vi "REPORT.init test.vi"(10 "Test OUT 2":T1={"Config HW"={"VISA Rigol DP832"="USB0::0x1AB1::0x0E11::DP8C191500901::INSTR", "Config Rigol DP832"=[{"Channel"=0, "V Limit"=5.5, "I Limit"=0.5, "V Out"=5.0}, {"Channel"=1, "V Limit"=5.5, "I Limit"=0.8, "V Out"=5.0}, {"Channel"=2, "V Limit"=5.5, "I Limit"=0.2, "V Out"=0.0}], "CTA Test#"="CTA013 A", "FT_Handle"=432866568, "Espera acceso FT"=10, "VISA Tek MDO3104"="Rigol_DP832", "VISA Key 81160A"="Rigol_DP832"}, "Config Test"=[{"Vasic"=2.8, "Global Reset"=FALSE, "Test Register?"=FALSE, "Test ADC?"=FALSE, "Test ADC"={"Repeats ADC"=100, "Max Desviation"=0.1}, "Limits ADC"={"Low"=[1.9, 1.3, 0.65, 0.0, 1.6, 1.4, 1.4, 0.9, 2.1, 0.85, 1.9], "High"=[2.1, 1.5, 0.85, 0.1, 1.4, 1.2, 1.2, 0.7, 1.9, 0.65, 1.7]}, "Test Max PN Min NP?"=FALSE, "Limits Max PN Min NP"={"Max P Upper"=2.177000045776367, "Min P Upper"=1.474, "Max N Upper"=1.475, "Min N Upper"=0.818, "Max P Lower"=1.888, "Min P Lower "=1.321, "Max N Lower"=1.322, "Min N Lower"=0.73}, "Test Rate Scan?"=FALSE, "Vin Rate Scan"=[], "Limits Rate Scan"={"High"=[0.15, 0.242, 0.331, 0.425, 0.512, 0.6, 0.688, 0.774, 0.847, 0.91], "Low"=[0.021, 0.11, 0.189, 0.27, 0.347, 0.421, 0.487, 0.551, 0.601, 0.635]}, "Test Rate Scan Adders?"=FALSE, "Vin Rate Adders"=[], "Limits Rate Scan adders"={"High"=[], "Low"=[]}, "Test offset analog?"=FALSE, "Lim Offset Analog"={"Max Analog"=0.05, "Min Analog"=-0.05}, "Test offset digital?"=FALSE, "Lim offset Dig"={"Max Dig"=0.05}, "Vasic real f.a."=2.8, "IBIAS"=FALSE, "VALUE IBIAS"=63}, {"Vasic"=2.8, "Global Reset"=FALSE, "Test Register?"=FALSE, "Test ADC?"=FALSE, "Test ADC"={"Repeats ADC"=100, "Max Desviation"=0.1}, "Limits ADC"={"Low"=[1.9, 1.3, 0.65, 0.0, 1.6, 1.4, 1.4, 0.9, 2.1, 0.85, 1.9], "High"=[2.1, 1.5, 0.85, 0.1, 1.4, 1.2, 1.2, 0.7, 1.9, 0.65, 1.7]}, "Test Max PN Min NP?"=FALSE, "Limits Max PN Min NP"={"Max P Upper"=2.177000045776367, "Min P Upper"=1.474, "Max N Upper"=1.475, "Min N Upper"=0.818, "Max P Lower"=1.888, "Min P Lower "=1.321, "Max N Lower"=1.322, "Min N Lower"=0.73}, "Test Rate Scan?"=FALSE, "Vin Rate Scan"=[], "Limits Rate Scan"={"High"=[0.15, 0.242, 0.331, 0.425, 0.512, 0.6, 0.688, 0.774, 0.847, 0.91], "Low"=[0.021, 0.11, 0.189, 0.27, 0.347, 0.421, 0.487, 0.551, 0.601, 0.635]}, "Test Rate Scan Adders?"=FALSE, "Vin Rate Adders"=[], "Limits Rate Scan adders"={"High"=[], "Low"=[]}, "Test offset analog?"=FALSE, "Lim Offset Analog"={"Max Analog"=0.05, "Min Analog"=-0.05}, "Test offset digital?"=FALSE, "Lim offset Dig"={"Max Dig"=0.05}, "Vasic real f.a."=2.8, "IBIAS"=FALSE, "VALUE IBIAS"=63}, {"Vasic"=2.8, "Global Reset"=FALSE, "Test Register?"=FALSE, "Test ADC?"=FALSE, "Test ADC"={"Repeats ADC"=100, "Max Desviation"=0.1}, "Limits ADC"={"Low"=[1.9, 1.3, 0.65, 0.0, 1.6, 1.4, 1.4, 0.9, 2.1, 0.85, 1.9], "High"=[2.1, 1.5, 0.85, 0.1, 1.4, 1.2, 1.2, 0.7, 1.9, 0.65, 1.7]}, "Test Max PN Min NP?"=FALSE, "Limits Max PN Min NP"={"Max P Upper"=2.177000045776367, "Min P Upper"=1.474, "Max N Upper"=1.475, "Min N Upper"=0.818, "Max P Lower"=1.888, "Min P Lower "=1.321, "Max N Lower"=1.322, "Min N Lower"=0.73}, "Test Rate Scan?"=FALSE, "Vin Rate Scan"=[], "Limits Rate Scan"={"High"=[0.15, 0.242, 0.331, 0.425, 0.512, 0.6, 0.688, 0.774, 0.847, 0.91], "Low"=[0.021, 0.11, 0.189, 0.27, 0.347, 0.421, 0.487, 0.551, 0.601, 0.635]}, "Test Rate Scan Adders?"=FALSE, "Vin Rate Adders"=[], "Limits Rate Scan adders"={"High"=[], "Low"=[]}, "Test offset analog?"=FALSE, "Lim Offset Analog"={"Max Analog"=0.05, "Min Analog"=-0.05}, "Test offset digital?"=FALSE, "Lim offset Dig"={"Max Dig"=0.05}, "Vasic real f.a."=2.8, "IBIAS"=FALSE, "VALUE IBIAS"=63}, {"Vasic"=2.8, "Global Reset"=FALSE, "Test Register?"=FALSE, "Test ADC?"=FALSE, "Test ADC"={"Repeats ADC"=100, "Max Desviation"=0.1}, "Limits ADC"={"Low"=[1.9, 1.3, 0.65, 0.0, 1.6, 1.4, 1.4, 0.9, 2.1, 0.85, 1.9], "High"=[2.1, 1.5, 0.85, 0.1, 1.4, 1.2, 1.2, 0.7, 1.9, 0.65, 1.7]}, "Test Max PN Min NP?"=FALSE, "Limits Max PN Min NP"={"Max P Upper"=2.177000045776367, "Min P Upper"=1.474, "Max N Upper"=1.475, "Min N Upper"=0.818, "Max P Lower"=1.888, "Min P Lower "=1.321, "Max N Lower"=1.322, "Min N Lower"=0.73}, "Test Rate Scan?"=FALSE, "Vin Rate Scan"=[], "Limits Rate Scan"={"High"=[0.15, 0.242, 0.331, 0.425, 0.512, 0.6, 0.688, 0.774, 0.847, 0.91], "Low"=[0.021, 0.11, 0.189, 0.27, 0.347, 0.421, 0.487, 0.551, 0.601, 0.635]}, "Test Rate Scan Adders?"=FALSE, "Vin Rate Adders"=[], "Limits Rate Scan adders"={"High"=[], "Low"=[]}, "Test offset analog?"=FALSE, "Lim Offset Analog"={"Max Analog"=0.05, "Min Analog"=-0.05}, "Test offset digital?"=FALSE, "Lim offset Dig"={"Max Dig"=0.05}, "Vasic real f.a."=2.8, "IBIAS"=FALSE, "VALUE IBIAS"=63}], "Result"=[{"Vasic Volt"=0, "Test Registros"={"Default Register OK"=FALSE, "Pattern Default"=[], "Read Default"=[], "W/R Register OK"=FALSE, "Pattern W/R"=[], "Read W/R"=[]}, "Test Dacs"={"Desviacion OK"=FALSE, "Means"=[], "Deviations"=[], "Desviations OK"=[], "Means OK"=[], "Graph Histogram"=[]}, "Test Max-Min PN"={"Max P Mini N OK"=FALSE, "PTHT Max P Min N"=[], "PTHT Max P Min N OK"=[], "NTHT Max P Min N"=[], "NTHT Max P Min N OK"=[], "Min P Max N OK"=FALSE, "PTHT Max N Min P"=[], "PTHT Max N Min P OK"=[], "NTHT Max N Min P"=[], "NTHT Max N Min P OK"=[], "Ref"=[]}, "Test Rate Scan"={"Rate Scan OK"=FALSE, "DAC TH0,TH1,TH2"=[], "Volt HLTH"=[], "Rate HLTH OK"=[], "DAC TH3,TH4,TH5"=[], "Volt LLTH"=[], "Rate LLTH 2 OK"=[], "Scaler 0"=[], "Ref"=[], "OFFSET HLTH"=[], "OFFSET LLTH"=[], "Real Voltage"=[]}, "Test Rate Scan adders"={"Rate Scan Adders OK"=FALSE, "DAC TH0,TH1,TH2"=[], "Volt HLTH"=[], "Add HLTH OK"=[], "DAC TH3,TH4,TH5"=[], "Volt LLTH"=[], "Add LLTH 2 OK"=[], "Scaler 0"=[], "Ref"=[], "OFFSET HLTH"=[], "OFFSET LLTH"=[], "Real Voltage"=[]}, "Test Offset Analog"={"Offset Analog OK"=FALSE, "V ADDOUT"=[], "Offset OK"=[], "Ref"=[]}, "Test Offset Digital"={"Offset Digital OK"=FALSE, "SCALER 1 START"=[], "SCALER 1 STOP"=[], "THX START"=[], "THX STOP"=[], "VHLTH START"=[], "VHLTH STOP"=[], "Index 1 Start"=[], "index 1 Stop"=[], "SCALER 2 START"=[], "SCALER 2 STOP"=[], "THX+3 START"=[], "THX+3 STOP"=[], "VLLTH START"=[], "VLLTH STOP"=[], "Index 2 Start"=[], "index 2 Stop"=[], "Dig HLTH OK"=[], "Dig LLTH 2 OK"=[], "Ref"=[]}, "info hardware"={"Iout V1"=0.0, "Iout V2"=0.0, "Iout V3"=0.0, "Vout V1"=0.0, "Vout V2"=0.0, "Vout V3"=0.0, "Temp"=0.0}, "Test Offset Analog add"={"Offset Analog add OK"=FALSE, "V ADDOUT add"=[], "Offset add OK"=[], "Ref add"=[]}, "info temp"={"T Asic Registers"=0.0, "T Board Test. ADC"=0.0, "T Asic Max Min N P"=0.0, "T Adc count"=0.0, "T Asic Digital Offset"=0.0, "T Asic Analog Offset"=0.0, "T Asic Analog add"=0.0, "T Asic Rate Scan"=0.0, "T Asic Rate Scan Adders"=0.0, "T Final"=0.0}}, {"Vasic Volt"=0, "Test Registros"={"Default Register OK"=FALSE, "Pattern Default"=[], "Read Default"=[], "W/R Register OK"=FALSE, "Pattern W/R"=[], "Read W/R"=[]}, "Test Dacs"={"Desviacion OK"=FALSE, "Means"=[], "Deviations"=[], "Desviations OK"=[], "Means OK"=[], "Graph Histogram"=[]}, "Test Max-Min PN"={"Max P Mini N OK"=FALSE, "PTHT Max P Min N"=[], "PTHT Max P Min N OK"=[], "NTHT Max P Min N"=[], "NTHT Max P Min N OK"=[], "Min P Max N OK"=FALSE, "PTHT Max N Min P"=[], "PTHT Max N Min P OK"=[], "NTHT Max N Min P"=[], "NTHT Max N Min P OK"=[], "Ref"=[]}, "Test Rate Scan"={"Rate Scan OK"=FALSE, "DAC TH0,TH1,TH2"=[], "Volt HLTH"=[], "Rate HLTH OK"=[], "DAC TH3,TH4,TH5"=[], "Volt LLTH"=[], "Rate LLTH 2 OK"=[], "Scaler 0"=[], "Ref"=[], "OFFSET HLTH"=[], "OFFSET LLTH"=[], "Real Voltage"=[]}, "Test Rate Scan adders"={"Rate Scan Adders OK"=FALSE, "DAC TH0,TH1,TH2"=[], "Volt HLTH"=[], "Add HLTH OK"=[], "DAC TH3,TH4,TH5"=[], "Volt LLTH"=[], "Add LLTH 2 OK"=[], "Scaler 0"=[], "Ref"=[], "OFFSET HLTH"=[], "OFFSET LLTH"=[], "Real Voltage"=[]}, "Test Offset Analog"={"Offset Analog OK"=FALSE, "V ADDOUT"=[], "Offset OK"=[], "Ref"=[]}, "Test Offset Digital"={"Offset Digital OK"=FALSE, "SCALER 1 START"=[], "SCALER 1 STOP"=[], "THX START"=[], "THX STOP"=[], "VHLTH START"=[], "VHLTH STOP"=[], "Index 1 Start"=[], "index 1 Stop"=[], "SCALER 2 START"=[], "SCALER 2 STOP"=[], "THX+3 START"=[], "THX+3 STOP"=[], "VLLTH START"=[], "VLLTH STOP"=[], "Index 2 Start"=[], "index 2 Stop"=[], "Dig HLTH OK"=[], "Dig LLTH 2 OK"=[], "Ref"=[]}, "info hardware"={"Iout V1"=0.0, "Iout V2"=0.0, "Iout V3"=0.0, "Vout V1"=0.0, "Vout V2"=0.0, "Vout V3"=0.0, "Temp"=0.0}, "Test Offset Analog add"={"Offset Analog add OK"=FALSE, "V ADDOUT add"=[], "Offset add OK"=[], "Ref add"=[]}, "info temp"={"T Asic Registers"=0.0, "T Board Test. ADC"=0.0, "T Asic Max Min N P"=0.0, "T Adc count"=0.0, "T Asic Digital Offset"=0.0, "T Asic Analog Offset"=0.0, "T Asic Analog add"=0.0, "T Asic Rate Scan"=0.0, "T Asic Rate Scan Adders"=0.0, "T Final"=0.0}}, {"Vasic Volt"=0, "Test Registros"={"Default Register OK"=FALSE, "Pattern Default"=[], "Read Default"=[], "W/R Register OK"=FALSE, "Pattern W/R"=[], "Read W/R"=[]}, "Test Dacs"={"Desviacion OK"=FALSE, "Means"=[], "Deviations"=[], "Desviations OK"=[], "Means OK"=[], "Graph Histogram"=[]}, "Test Max-Min PN"={"Max P Mini N OK"=FALSE, "PTHT Max P Min N"=[], "PTHT Max P Min N OK"=[], "NTHT Max P Min N"=[], "NTHT Max P Min N OK"=[], "Min P Max N OK"=FALSE, "PTHT Max N Min P"=[], "PTHT Max N Min P OK"=[], "NTHT Max N Min P"=[], "NTHT Max N Min P OK"=[], "Ref"=[]}, "Test Rate Scan"={"Rate Scan OK"=FALSE, "DAC TH0,TH1,TH2"=[], "Volt HLTH"=[], "Rate HLTH OK"=[], "DAC TH3,TH4,TH5"=[], "Volt LLTH"=[], "Rate LLTH 2 OK"=[], "Scaler 0"=[], "Ref"=[], "OFFSET HLTH"=[], "OFFSET LLTH"=[], "Real Voltage"=[]}, "Test Rate Scan adders"={"Rate Scan Adders OK"=FALSE, "DAC TH0,TH1,TH2"=[], "Volt HLTH"=[], "Add HLTH OK"=[], "DAC TH3,TH4,TH5"=[], "Volt LLTH"=[], "Add LLTH 2 OK"=[], "Scaler 0"=[], "Ref"=[], "OFFSET HLTH"=[], "OFFSET LLTH"=[], "Real Voltage"=[]}, "Test Offset Analog"={"Offset Analog OK"=FALSE, "V ADDOUT"=[], "Offset OK"=[], "Ref"=[]}, "Test Offset Digital"={"Offset Digital OK"=FALSE, "SCALER 1 START"=[], "SCALER 1 STOP"=[], "THX START"=[], "THX STOP"=[], "VHLTH START"=[], "VHLTH STOP"=[], "Index 1 Start"=[], "index 1 Stop"=[], "SCALER 2 START"=[], "SCALER 2 STOP"=[], "THX+3 START"=[], "THX+3 STOP"=[], "VLLTH START"=[], "VLLTH STOP"=[], "Index 2 Start"=[], "index 2 Stop"=[], "Dig HLTH OK"=[], "Dig LLTH 2 OK"=[], "Ref"=[]}, "info hardware"={"Iout V1"=0.0, "Iout V2"=0.0, "Iout V3"=0.0, "Vout V1"=0.0, "Vout V2"=0.0, "Vout V3"=0.0, "Temp"=0.0}, "Test Offset Analog add"={"Offset Analog add OK"=FALSE, "V ADDOUT add"=[], "Offset add OK"=[], "Ref add"=[]}, "info temp"={"T Asic Registers"=0.0, "T Board Test. ADC"=0.0, "T Asic Max Min N P"=0.0, "T Adc count"=0.0, "T Asic Digital Offset"=0.0, "T Asic Analog Offset"=0.0, "T Asic Analog add"=0.0, "T Asic Rate Scan"=0.0, "T Asic Rate Scan Adders"=0.0, "T Final"=0.0}}, {"Vasic Volt"=0, "Test Registros"={"Default Register OK"=FALSE, "Pattern Default"=[], "Read Default"=[], "W/R Register OK"=FALSE, "Pattern W/R"=[], "Read W/R"=[]}, "Test Dacs"={"Desviacion OK"=FALSE, "Means"=[], "Deviations"=[], "Desviations OK"=[], "Means OK"=[], "Graph Histogram"=[]}, "Test Max-Min PN"={"Max P Mini N OK"=FALSE, "PTHT Max P Min N"=[], "PTHT Max P Min N OK"=[], "NTHT Max P Min N"=[], "NTHT Max P Min N OK"=[], "Min P Max N OK"=FALSE, "PTHT Max N Min P"=[], "PTHT Max N Min P OK"=[], "NTHT Max N Min P"=[], "NTHT Max N Min P OK"=[], "Ref"=[]}, "Test Rate Scan"={"Rate Scan OK"=FALSE, "DAC TH0,TH1,TH2"=[], "Volt HLTH"=[], "Rate HLTH OK"=[], "DAC TH3,TH4,TH5"=[], "Volt LLTH"=[], "Rate LLTH 2 OK"=[], "Scaler 0"=[], "Ref"=[], "OFFSET HLTH"=[], "OFFSET LLTH"=[], "Real Voltage"=[]}, "Test Rate Scan adders"={"Rate Scan Adders OK"=FALSE, "DAC TH0,TH1,TH2"=[], "Volt HLTH"=[], "Add HLTH OK"=[], "DAC TH3,TH4,TH5"=[], "Volt LLTH"=[], "Add LLTH 2 OK"=[], "Scaler 0"=[], "Ref"=[], "OFFSET HLTH"=[], "OFFSET LLTH"=[], "Real Voltage"=[]}, "Test Offset Analog"={"Offset Analog OK"=FALSE, "V ADDOUT"=[], "Offset OK"=[], "Ref"=[]}, "Test Offset Digital"={"Offset Digital OK"=FALSE, "SCALER 1 START"=[], "SCALER 1 STOP"=[], "THX START"=[], "THX STOP"=[], "VHLTH START"=[], "VHLTH STOP"=[], "Index 1 Start"=[], "index 1 Stop"=[], "SCALER 2 START"=[], "SCALER 2 STOP"=[], "THX+3 START"=[], "THX+3 STOP"=[], "VLLTH START"=[], "VLLTH STOP"=[], "Index 2 Start"=[], "index 2 Stop"=[], "Dig HLTH OK"=[], "Dig LLTH 2 OK"=[], "Ref"=[]}, "info hardware"={"Iout V1"=0.0, "Iout V2"=0.0, "Iout V3"=0.0, "Vout V1"=0.0, "Vout V2"=0.0, "Vout V3"=0.0, "Temp"=0.0}, "Test Offset Analog add"={"Offset Analog add OK"=FALSE, "V ADDOUT add"=[], "Offset add OK"=[], "Ref add"=[]}, "info temp"={"T Asic Registers"=0.0, "T Board Test. ADC"=0.0, "T Asic Max Min N P"=0.0, "T Adc count"=0.0, "T Asic Digital Offset"=0.0, "T Asic Analog Offset"=0.0, "T Asic Analog add"=0.0, "T Asic Rate Scan"=0.0, "T Asic Rate Scan Adders"=0.0, "T Final"=0.0}}], "Execucion Test"={"Vasic Actual"=0}, "Config VGA"={"Theoretical Voltage"=[0.1, 0.2, 0.3, 0.4, 0.5, 0.6, 0.7, 0.8, 0.9, 1.0], "Real Voltage"=[0.10285, 0.20714, 0.29957, 0.40485, 0.49571, 0.60685, 0.69771, 0.80114, 0.89714, 0.99885], "Pulse Width"=57344, "Frecuency Pulse"=1000000.0, "VGA Gain"=[9, 16, 24, 34, 43, 52, 61, 72, 81, 93]}, "Test Info"={"Asic"="", "Operator"="", "Place"="", "Time start"=timestamp(0 s since 1904-01-01), "Time stop"=timestamp(0 s since 1904-01-01)}, "Info machine"={"SO"="", "SO Name"="", "SO Ver"="", "SO Build"="", "CPU"="", "APP"="", "APP YEAR"="", "APP ver"="", "APP User"="", "APP Serail"="", "MAC"=[], "PC NAME"=[], "PC IP"=[], "BIOS MANU"="", "BIOS NAME"="", "BIOS SERIAL"="", "BOARD MANU"="", "BOARD NAME"="", "BOARD SERIAL"="", "Driver Version"="", "Library Version"="", "FPGA Ver"=0, "ID CTA board"=0, "LAST BOOT"="", "LABVIEW Ver"=0}, "Partial Report"="", "CONFIG GEN"=[]} {"CONFIG GEN"."Vasic Theorical" min=1.0 max=1000000.0 step=1.0 format="%#_6pV"; "CONFIG GEN"."Frequency" min=0.001 max=333000000.0 step=1000.0 format="%#_6pHz"; "CONFIG GEN"."Leading Edge Time" min=1e-09 max=1.0 step=1e-10 format="%#_6ps"; "CONFIG GEN"."Trailing Edge Time" min=1e-09 max=1.0 step=1e-10 format="%#_6ps"; "CONFIG GEN"."Delay" min=0.0 max=1.0 step=1e-12 format="%#_6ps"; "CONFIG GEN"."Trigger Level Sync" items=["ECL", "TTL"]; "CONFIG GEN"."Trigger Sync Out" items=["AB"=3, "B"=2, "A"=1, "None"=0]; "CONFIG GEN"."Load" min=1.0 max=1000000.0 step=1.0 format="%#_6p"; "CONFIG GEN"."DC Offset" min=-10.0 max=10.0 step=0.1 format="%#_6pV"; "CONFIG GEN"."Amplitude" min=0.05 max=5.0 step=0.001 format="%#_6pV"; "CONFIG GEN"."Width Time" min=1.5e-09 max=1.0 step=1e-10 format="%#_6ps"; "CONFIG GEN"."Channel" items=["Channel1"=1, "Channel2"=2]; "Config VGA"."Theoretical Voltage" format="%1.4f"; "Config VGA"."VGA Gain" format="%02x"; "Config VGA"."Frecuency Pulse" format="%0_2p"; "Config VGA"."Pulse Width" format="%04x"; "Config VGA"."Real Voltage" format="%1.5f"; "Config Test"."VALUE IBIAS" max=63 step=1; "Config Test"."Vasic real f.a." min=2.8 max=3.8 step=0.01 format="%.2g"; "Config Test"."Limits Rate Scan adders"."Low" format="%1.3f"; "Config Test"."Limits Rate Scan adders"."High" format="%1.3f"; "Config Test"."Limits ADC"."High" format="%1.4f"; "Config Test"."Limits ADC"."Low" format="%1.3f"; "Config Test"."Lim offset Dig"."Max Dig" format="%.3g"; "Config Test"."Lim Offset Analog"."Min Analog" format="%.3g"; "Config Test"."Lim Offset Analog"."Max Analog" format="%.3g"; "Config Test"."Limits Rate Scan"."Low" format="%1.4f"; "Config Test"."Limits Rate Scan"."High" format="%1.3f"; "Config Test"."Limits Max PN Min NP"."Min P Upper" format="%.3g"; "Config Test"."Limits Max PN Min NP"."Min P Lower" format="%.3g"; "Config Test"."Limits Max PN Min NP"."Max N Lower" format="%.3g"; "Config Test"."Limits Max PN Min NP"."Max N Upper" format="%.3g"; "Config Test"."Limits Max PN Min NP"."Min N Lower" format="%.3g"; "Config Test"."Limits Max PN Min NP"."Min N Upper" format="%.3g"; "Config Test"."Limits Max PN Min NP"."Max P Upper" format="%.3g"; "Config Test"."Limits Max PN Min NP"."Max P Lower" format="%.3g"; "Config Test"."Vasic" min=2.8 max=3.8 step=0.01 format="%.2g"; "Config HW"."Config Rigol DP832"."Channel" items=["+30V Channel 1", "+30V Channel 2", "+5V Channel 3"]; "Config HW"."Config Rigol DP832"."V Limit" format="%.1g"; "Config HW"."Config Rigol DP832"."I Limit" format="%.1g"; "Config HW"."Config Rigol DP832"."V Out" format="%.1g"; "Result"."Test Registros"."Read W/R" format="%04x"; "Result"."Test Registros"."Pattern W/R" format="%04x"; "Result"."Test Registros"."Read Default" format="%04x"; "Result"."Test Registros"."Pattern Default" format="%04x"}, 11 "Text In":string) -> (1 "OK, Fault":string, 2 "OK, Fault 2":bool, 3 "Text Out":string)   [LabVIEW 2019]
uses:
  Test.ctl
  TEST.TEST CONFIG HW.ctl
  Rigol DP832/DP832_Control Channels.ctl
  TEST.TEST CONFIG TEST MATRIZ.ctl
  TEST.TEST CONFIG TEST.ctl
  TEST.TEST RESULT.ctl
  test_result fvasic.ctl
  TEST.TEST EXECUTION TEST.ctl
  TEST.TEST CONFIG VGA.ctl
  TEST.TEST TEST INFO.ctl
  TEST.TEST INFO PC.ctl
  GenPulse_configurar.ctl
panel:
  # "Modo 2\nModo 3\nModo 4\nModo 2\nModo 3\nModo 4"
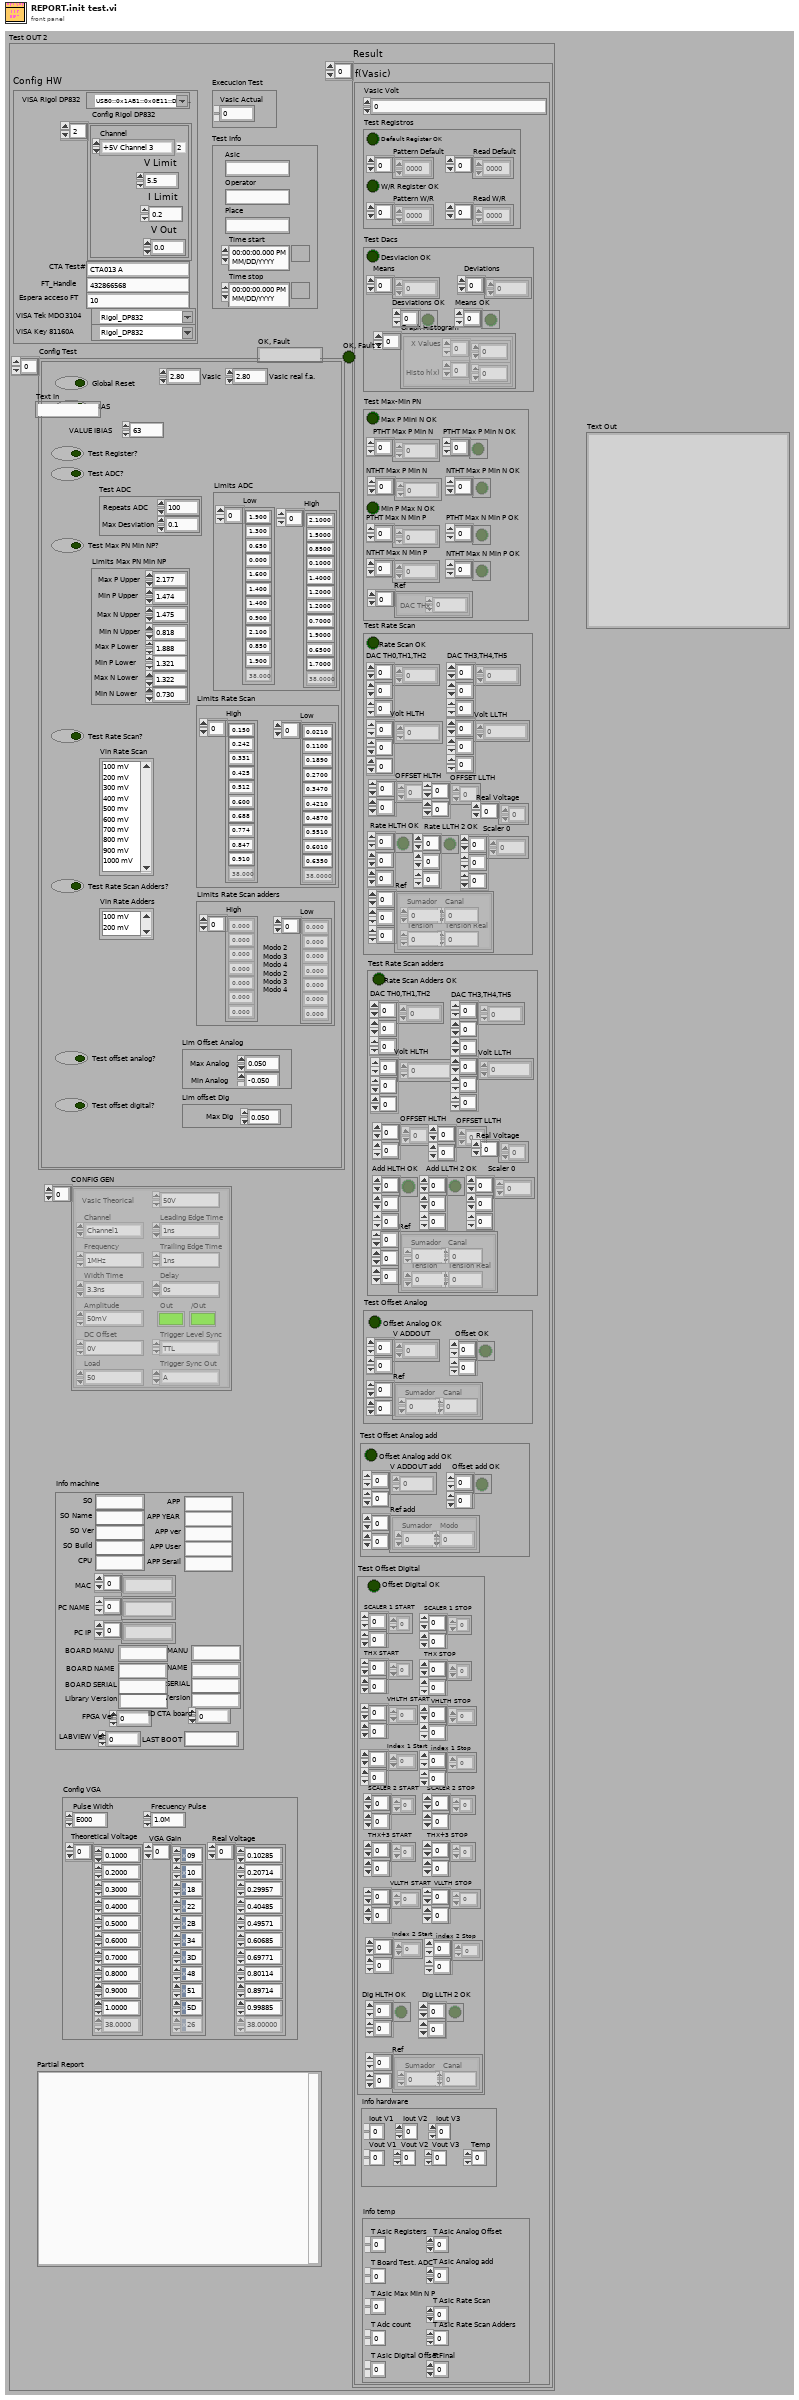
[diagram p1: front panel]
types:
  T1 = typedef "Test.ctl" = cluster{"Config HW":T2, "Config Test":T4, "Result":T6, "Execucion Test":T8, "Config VGA":T9, "Test Info":T10, "Info machine":T11, "Partial Report":string, "CONFIG GEN":T12[]}
  T2 = typedef "TEST.TEST CONFIG HW.ctl" = cluster{"VISA Rigol DP832":refnum<visa-resource-name>, "Config Rigol DP832":cluster{"Channel":T3, "V Limit":dbl, "I Limit":dbl, "V Out":dbl}[], "CTA Test#":string, "FT_Handle":u32, "Espera acceso FT":u32, "VISA Tek MDO3104":refnum<visa-resource-name>, "VISA Key 81160A":refnum<visa-resource-name>}
  T3 = typedef "DP832_Control Channels.ctl" = i32
  T4 = typedef "TEST.TEST CONFIG TEST MATRIZ.ctl" = T5[]
  T5 = typedef "TEST.TEST CONFIG TEST.ctl" = cluster{"Vasic":dbl, "Global Reset":bool, "Test Register?":bool, "Test ADC?":bool, "Test ADC":cluster{"Repeats ADC":i32, "Max Desviation":dbl}, "Limits ADC":cluster{"Low":dbl[], "High":dbl[]}, "Test Max PN Min NP?":bool, "Limits Max PN Min NP":cluster{"Max P Upper":dbl, "Min P Upper":dbl, "Max N Upper":dbl, "Min N Upper":dbl, "Max P Lower":dbl, "Min P Lower ":dbl, "Max N Lower":dbl, "Min N Lower":dbl}, "Test Rate Scan?":bool, "Vin Rate Scan":i32[], "Limits Rate Scan":cluster{"High":dbl[], "Low":dbl[]}, "Test Rate Scan Adders?":bool, "Vin Rate Adders":i32[], "Limits Rate Scan adders":cluster{"High":dbl[], "Low":dbl[]}, "Test offset analog?":bool, "Lim Offset Analog":cluster{"Max Analog":dbl, "Min Analog":dbl}, "Test offset digital?":bool, "Lim offset Dig":cluster{"Max Dig":dbl}, "Vasic real f.a.":dbl, "IBIAS":bool, "VALUE IBIAS":u8}
  T6 = typedef "TEST.TEST RESULT.ctl" = T7[]
  T7 = typedef "test_result fvasic.ctl" = cluster{"Vasic Volt":i32, "Test Registros":cluster{"Default Register OK":bool, "Pattern Default":u16[], "Read Default":u16[], "W/R Register OK":bool, "Pattern W/R":u16[], "Read W/R":u16[]}, "Test Dacs":cluster{"Desviacion OK":bool, "Means":dbl[], "Deviations":dbl[], "Desviations OK":bool[], "Means OK":bool[], "Graph Histogram":cluster{"X Values":dbl[], "Histo h(x)":i32[]}[]}, "Test Max-Min PN":cluster{"Max P Mini N OK":bool, "PTHT Max P Min N":dbl[], "PTHT Max P Min N OK":bool[], "NTHT Max P Min N":dbl[], "NTHT Max P Min N OK":bool[], "Min P Max N OK":bool, "PTHT Max N Min P":dbl[], "PTHT Max N Min P OK":bool[], "NTHT Max N Min P":dbl[], "NTHT Max N Min P OK":bool[], "Ref":cluster{"DAC THx":u8}[]}, "Test Rate Scan":cluster{"Rate Scan OK":bool, "DAC TH0,TH1,TH2":u16[][][], "Volt HLTH":dbl[][][], "Rate HLTH OK":bool[][][], "DAC TH3,TH4,TH5":u16[][][], "Volt LLTH":dbl[][][], "Rate LLTH 2 OK":bool[][][], "Scaler 0":u16[][][], "Ref":cluster{"Sumador":u8, "Canal":u8, "Tension":u8, "Tension Real":dbl}[][][], "OFFSET HLTH":dbl[][], "OFFSET LLTH":dbl[][], "Real Voltage":dbl[]}, "Test Rate Scan adders":cluster{"Rate Scan Adders OK":bool, "DAC TH0,TH1,TH2":u16[][][], "Volt HLTH":dbl[][][], "Add HLTH OK":bool[][][], "DAC TH3,TH4,TH5":u16[][][], "Volt LLTH":dbl[][][], "Add LLTH 2 OK":bool[][][], "Scaler 0":u16[][][], "Ref":cluster{"Sumador":u8, "Canal":u8, "Tension":u8, "Tension Real":dbl}[][][], "OFFSET HLTH":dbl[][], "OFFSET LLTH":dbl[][], "Real Voltage":dbl[]}, "Test Offset Analog":cluster{"Offset Analog OK":bool, "V ADDOUT":dbl[][], "Offset OK":bool[][], "Ref":cluster{"Sumador":u8, "Canal":u8}[][]}, "Test Offset Digital":cluster{"Offset Digital OK":bool, "SCALER 1 START":u16[][], "SCALER 1 STOP":u16[][], "THX START":u16[][], "THX STOP":u16[][], "VHLTH START":dbl[][], "VHLTH STOP":dbl[][], "Index 1 Start":i32[][], "index 1 Stop":i32[][], "SCALER 2 START":u16[][], "SCALER 2 STOP":u16[][], "THX+3 START":u16[][], "THX+3 STOP":u16[][], "VLLTH START":dbl[][], "VLLTH STOP":dbl[][], "Index 2 Start":i32[][], "index 2 Stop":i32[][], "Dig HLTH OK":bool[][], "Dig LLTH 2 OK":bool[][], "Ref":cluster{"Sumador":u8, "Canal":u8}[][]}, "info hardware":cluster{"Iout V1":dbl, "Iout V2":dbl, "Iout V3":dbl, "Vout V1":dbl, "Vout V2":dbl, "Vout V3":dbl, "Temp":dbl}, "Test Offset Analog add":cluster{"Offset Analog add OK":bool, "V ADDOUT add":dbl[][], "Offset add OK":bool[][], "Ref add":cluster{"Sumador":u8, "Modo":u8}[][]}, "info temp":cluster{"T Asic Registers":dbl, "T Board Test. ADC":dbl, "T Asic Max Min N P":dbl, "T Adc count":dbl, "T Asic Digital Offset":dbl, "T Asic Analog Offset":dbl, "T Asic Analog add":dbl, "T Asic Rate Scan":dbl, "T Asic Rate Scan Adders":dbl, "T Final":dbl}}
  T8 = typedef "TEST.TEST EXECUTION TEST.ctl" = cluster{"Vasic Actual":i32}
  T9 = typedef "TEST.TEST CONFIG VGA.ctl" = cluster{"Theoretical Voltage":dbl[], "Real Voltage":dbl[], "Pulse Width":u16, "Frecuency Pulse":dbl, "VGA Gain":u8[]}
  T10 = typedef "TEST.TEST TEST INFO.ctl" = cluster{"Asic":string, "Operator":string, "Place":string, "Time start":timestamp, "Time stop":timestamp}
  T11 = typedef "TEST.TEST INFO PC.ctl" = cluster{"SO":string, "SO Name":string, "SO Ver":string, "SO Build":string, "CPU":string, "APP":string, "APP YEAR":string, "APP ver":string, "APP User":string, "APP Serail":string, "MAC":string[], "PC NAME":string[], "PC IP":string[], "BIOS MANU":string, "BIOS NAME":string, "BIOS SERIAL":string, "BOARD MANU":string, "BOARD NAME":string, "BOARD SERIAL":string, "Driver Version":string, "Library Version":string, "FPGA Ver":u8, "ID CTA board":u64, "LAST BOOT":string, "LABVIEW Ver":u32}
  T12 = typedef "GenPulse_configurar.ctl" = cluster{"Channel":u16, "Frequency":dbl, "Width Time":dbl, "Amplitude":dbl, "DC Offset":dbl, "Load":dbl, "Leading Edge Time":dbl, "Trailing Edge Time":dbl, "Delay":dbl, "Out":bool, "/Out":bool, "Trigger Level Sync":u16, "Trigger Sync Out":u16, "Vasic Theorical":dbl}
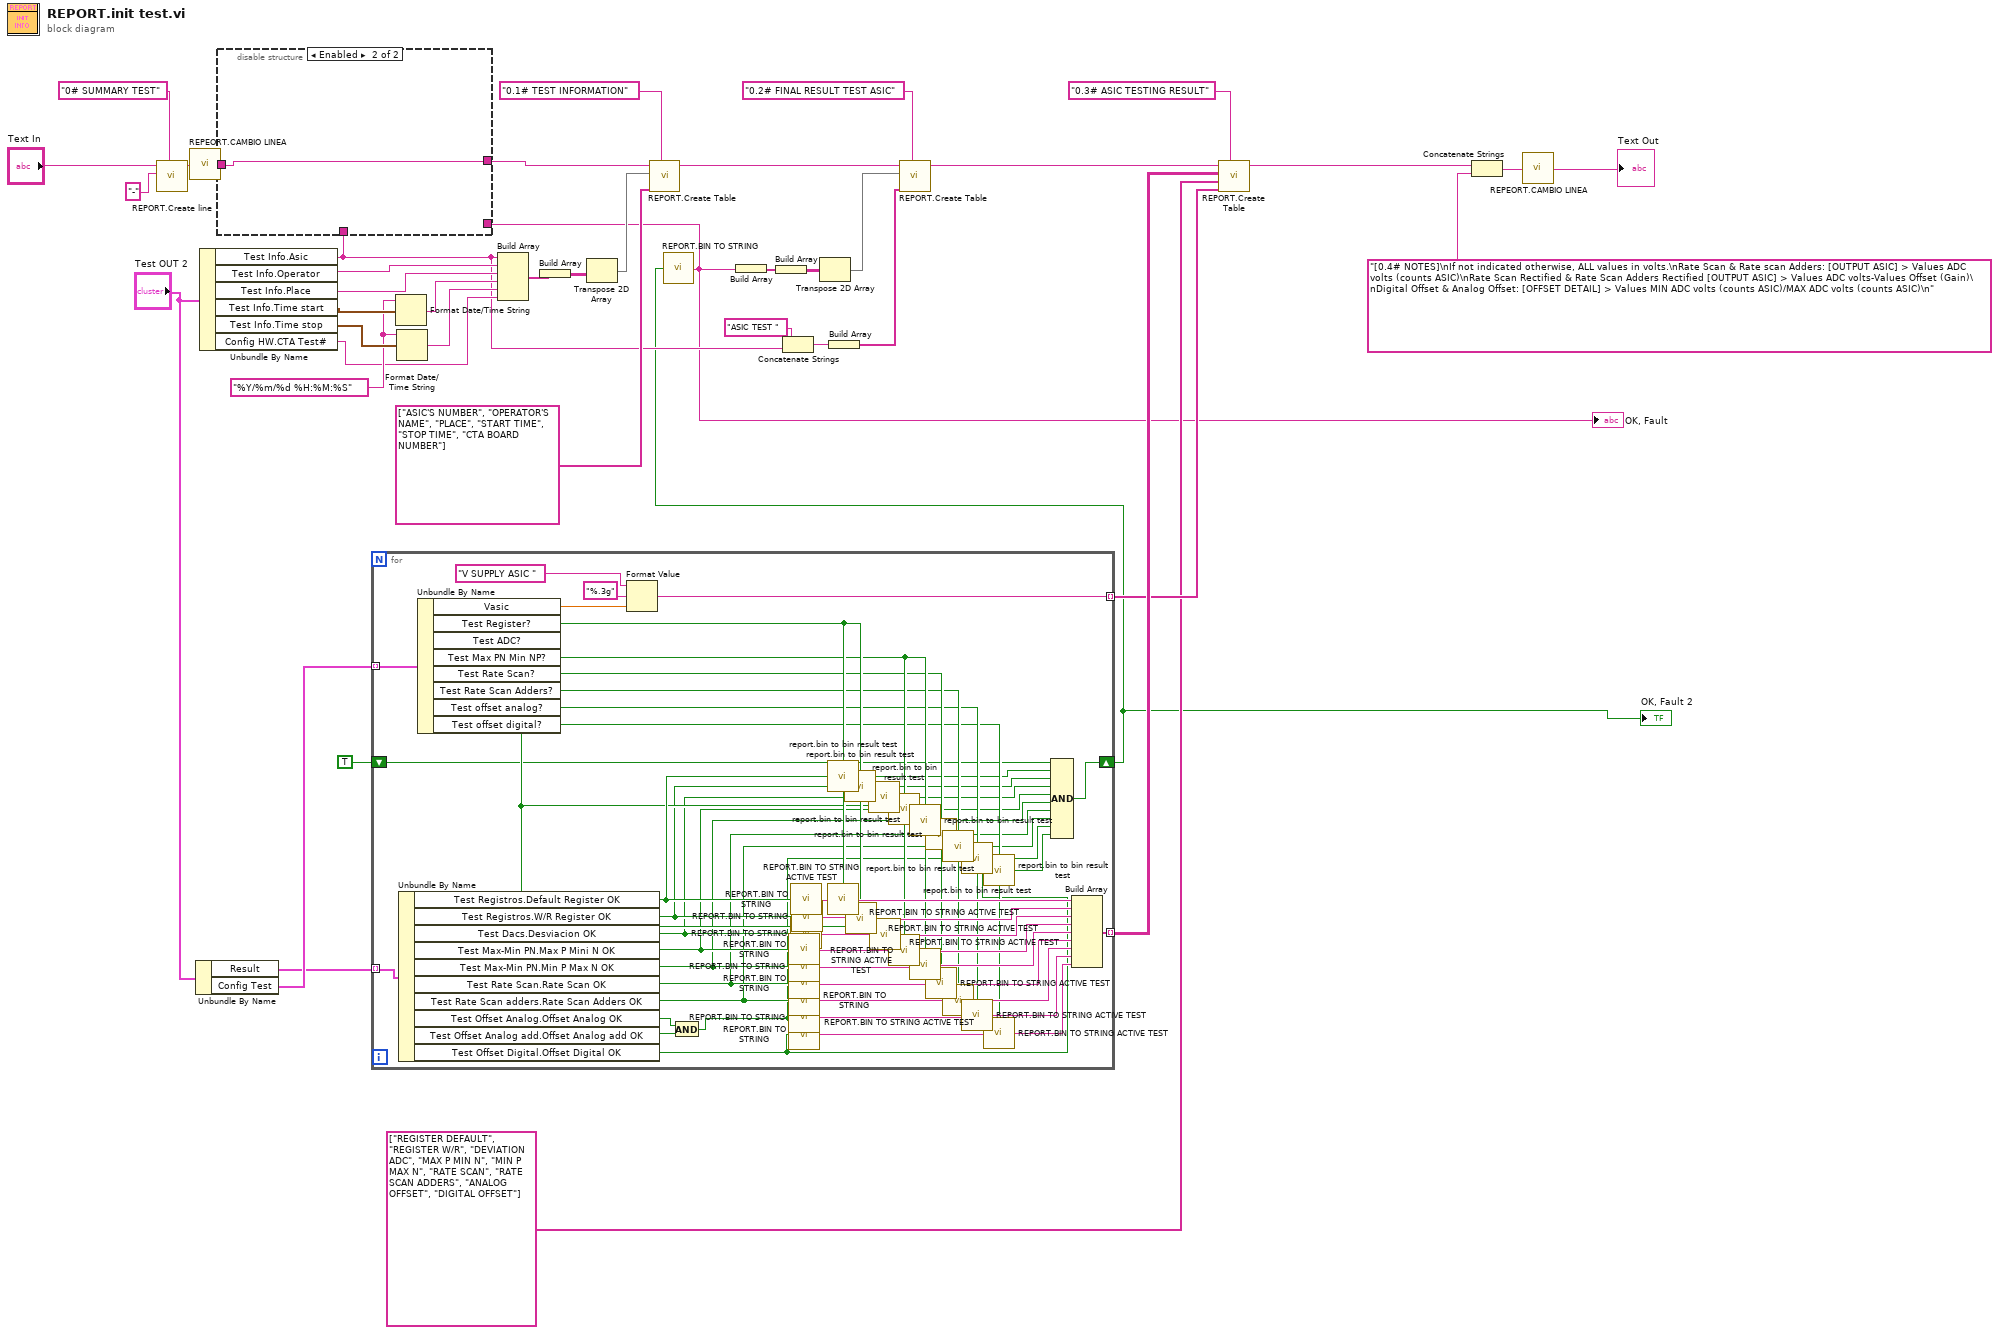
[diagram p0: block diagram]
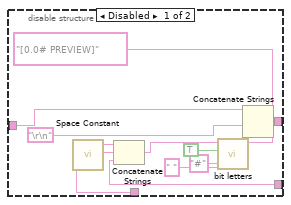
[diagram p2: hidden frame]
diagram:
  w38 = "%Y/%m/%d %H:%M:%S" ("time format string (%c)")
  n1 = call "REPORT.Create line.vi"("Secction"="0# SUMMARY TEST", "Char"="-", "Text In"="Text In") -> ("Text Out"=w28:string)  [unwired: 8 in]
  n2 = call "REPEORT.CAMBIO LINEA.vi"("Text Out"=w28) -> ("String"=w3:string)  [unwired: 8 in]
  n3 = Unbundle By Name("Test OUT 2") -> ("Result"=w22:T6, "Config Test"=w23:T4)
  n4 = Unbundle By Name("Test OUT 2") -> ("Test Info.Asic"=w5:string, "Test Info.Operator"=w37:string, "Test Info.Place"=w17:string, "Test Info.Time start"=w40:timestamp, "Test Info.Time stop"=w39:timestamp, "Config HW.CTA Test#"=w34:string)
  n5 = for {
    tunnel: w23 -> [w97] mode=indexing
    tunnel: [w94] -> w19 mode=indexing
    tunnel: w22 -> [w93] mode=indexing
    tunnel: [w73] -> w20 mode=indexing
    shift-right: [w49] -> w1
    shift-left: TRUE -> [w48]
    n6 = Unbundle By Name(w93) -> ("Test Registros.Default Register OK"=w72:bool, "Test Registros.W/R Register OK"=w64:bool, "Test Dacs.Desviacion OK"=w63:bool, "Test Max-Min PN.Max P Mini N OK"=w62:bool, "Test Max-Min PN.Min P Max N OK"=w61:bool, "Test Rate Scan.Rate Scan OK"=w60:bool, "Test Rate Scan adders.Rate Scan Adders OK"=w59:bool, "Test Offset Analog.Offset Analog OK"=w46:bool, "Test Offset Analog add.Offset Analog add OK"=w45:bool, "Test Offset Digital.Offset Digital OK"=w47:bool)
    n7 = Unbundle By Name(w97) -> ("Vasic"=w95:dbl, "Test Register?"=w71:bool, "Test ADC?"=w70:bool, "Test Max PN Min NP?"=w69:bool, "Test Rate Scan?"=w68:bool, "Test Rate Scan Adders?"=w67:bool, "Test offset analog?"=w66:bool, "Test offset digital?"=w65:bool)
    n8 = Format Value(string ("")="V SUPPLY ASIC " ("Date"), format string="%.3g", value (0)=w95) -> (output string=w94:string)
    n9 = And(x=w46, y=w45) -> (x .and. y?=w44:bool)
    n10 = call "REPORT.BIN TO STRING.vi"("Resultado test"=w62) -> ("OK, Fault"=w89:string)  [unwired: 14 in]
    n11 = call "REPORT.BIN TO STRING.vi"("Resultado test"=w61) -> ("OK, Fault"=w88:string)  [unwired: 14 in]
    n12 = call "REPORT.BIN TO STRING.vi"("Resultado test"=w60) -> ("OK, Fault"=w87:string)  [unwired: 14 in]
    n13 = call "REPORT.BIN TO STRING.vi"("Resultado test"=w59) -> ("OK, Fault"=w86:string)  [unwired: 14 in]
    n14 = call "REPORT.BIN TO STRING.vi"("Resultado test"=w44) -> ("OK, Fault"=w85:string)  [unwired: 14 in]
    n15 = call "REPORT.BIN TO STRING.vi"("Resultado test"=w47) -> ("OK, Fault"=w84:string)  [unwired: 14 in]
    n16 = call "REPORT.BIN TO STRING.vi"("Resultado test"=w72) -> ("OK, Fault"=w92:string)  [unwired: 14 in]
    n17 = call "REPORT.BIN TO STRING.vi"("Resultado test"=w63) -> ("OK, Fault"=w90:string)  [unwired: 14 in]
    n18 = call "REPORT.BIN TO STRING.vi"("Resultado test"=w64) -> ("OK, Fault"=w91:string)  [unwired: 14 in]
    n19 = call "report.bin to bin result test.vi"("Result test"=w72, "Test?"=w71) -> ("T= T test or No data"=w58:bool)  [unwired: 13 in]
    n20 = call "REPORT.BIN TO STRING ACTIVE TEST.vi"("realizar test?"=w71, "OK o Fault"=w92) -> ("(OK, Fault) (No data)"=w82:string)  [unwired: 13 in]
    n21 = call "report.bin to bin result test.vi"("Result test"=w64, "Test?"=w71) -> ("T= T test or No data"=w57:bool)  [unwired: 13 in]
    n22 = call "REPORT.BIN TO STRING ACTIVE TEST.vi"("realizar test?"=w71, "OK o Fault"=w91) -> ("(OK, Fault) (No data)"=w81:string)  [unwired: 13 in]
    n23 = call "report.bin to bin result test.vi"("Result test"=w63, "Test?"=w70) -> ("T= T test or No data"=w56:bool)  [unwired: 13 in]
    n24 = call "REPORT.BIN TO STRING ACTIVE TEST.vi"("realizar test?"=w70, "OK o Fault"=w90) -> ("(OK, Fault) (No data)"=w80:string)  [unwired: 13 in]
    n25 = call "report.bin to bin result test.vi"("Result test"=w62, "Test?"=w69) -> ("T= T test or No data"=w55:bool)  [unwired: 13 in]
    n26 = call "REPORT.BIN TO STRING ACTIVE TEST.vi"("realizar test?"=w69, "OK o Fault"=w89) -> ("(OK, Fault) (No data)"=w79:string)  [unwired: 13 in]
    n27 = call "report.bin to bin result test.vi"("Result test"=w61, "Test?"=w69) -> ("T= T test or No data"=w54:bool)  [unwired: 13 in]
    n28 = call "REPORT.BIN TO STRING ACTIVE TEST.vi"("realizar test?"=w69, "OK o Fault"=w88) -> ("(OK, Fault) (No data)"=w78:string)  [unwired: 13 in]
    n29 = call "report.bin to bin result test.vi"("Result test"=w60, "Test?"=w68) -> ("T= T test or No data"=w53:bool)  [unwired: 13 in]
    n30 = call "REPORT.BIN TO STRING ACTIVE TEST.vi"("realizar test?"=w68, "OK o Fault"=w87) -> ("(OK, Fault) (No data)"=w77:string)  [unwired: 13 in]
    n31 = call "report.bin to bin result test.vi"("Result test"=w59, "Test?"=w67) -> ("T= T test or No data"=w52:bool)  [unwired: 13 in]
    n32 = call "REPORT.BIN TO STRING ACTIVE TEST.vi"("realizar test?"=w67, "OK o Fault"=w86) -> ("(OK, Fault) (No data)"=w76:string)  [unwired: 13 in]
    n33 = call "report.bin to bin result test.vi"("Result test"=w44, "Test?"=w66) -> ("T= T test or No data"=w51:bool)  [unwired: 13 in]
    n34 = call "REPORT.BIN TO STRING ACTIVE TEST.vi"("realizar test?"=w66, "OK o Fault"=w85) -> ("(OK, Fault) (No data)"=w75:string)  [unwired: 13 in]
    n35 = call "report.bin to bin result test.vi"("Result test"=w47, "Test?"=w65) -> ("T= T test or No data"=w50:bool)  [unwired: 13 in]
    n36 = call "REPORT.BIN TO STRING ACTIVE TEST.vi"("realizar test?"=w65, "OK o Fault"=w84) -> ("(OK, Fault) (No data)"=w74:string)  [unwired: 13 in]
    n37 = Compound Arithmetic op=AND(w48, w58, w57, w56, w55, w54, w53, w52, w51, w50) -> (w49:bool)
    n38 = Build Array(w82, w81, w80, w79, w78, w77, w76, w75, w74) -> (w73:string[])
  }
  "OK, Fault 2" <- w1
  n39 = Format Date/Time String(time format string (%c)=w38, seconds (now)=w40) -> (date/time string=w36:string)  [unwired: 1 in]
  n40 = Format Date/Time String(time format string (%c)=w38, seconds (now)=w39) -> (date/time string=w35:string)  [unwired: 1 in]
  n41 = Build Array(w5, w37, w17, w36, w35, w34) -> (w33:string[])
  n42 = Build Array(w33) -> (w32:string[][])
  n43 = Transpose 2D Array(2D array=w32) -> (transposed array=w31:string[][])
  n44 = call "REPORT.BIN TO STRING.vi"("Resultado test"=w1) -> ("OK, Fault"=w4:string)  [unwired: 14 in]
  "OK, Fault" <- w4
  n45 = disable-structure shown="Enabled" {
    disable-tunnel: w5 -> [w109 _]
    disable-tunnel: w4 -> [w107 _]
    disable-tunnel: w3 -> [w100 w110]
    disable-tunnel: [w98 w110] -> w2
    frame Disabled {
      # "Mentes cortas"
      n46 = call <vilib>:"Space Constant.vi"() -> ("String"=w108:string)
      n47 = Concatenate Strings(w109, w108, w107) -> (w106:string)
      n48 = call "bit letters.vi"("String \"0\""=" " ("String \"0\""), "String \"1\""="#" ("String \"1\""), "Letras y string \"0\" / String \"1 y 0\""=TRUE ("Letras y string \"0\" / String \"1 y 0\""), "Texto"=w106) -> ("big letters"=w99:string)  [unwired: 7 in]
      n49 = Concatenate Strings(w100, "[0.0# PREVIEW]" ("Secction"), "\r\n", w99) -> (w98:string)
    }
    frame Enabled {
    }
  }
  n50 = call "REPORT.Create Table.vi"("Secction"="0.1# TEST INFORMATION", "Row Headers"=string[] ["ASIC'S NUMBER", "OPERATOR'S NAME", "PLACE", "START TIME", "STOP TIME", "CTA BOARD NUMBER"], "Text 2d"=w31, "Text In"=w2) -> ("Text Out"=w15:string)  [unwired: 4 in, 1 out]
  n51 = Build Array(w4) -> (w12:string[])
  n52 = Build Array(w12) -> (w11:string[][])
  n53 = Concatenate Strings("ASIC TEST " ("Date"), w5) -> (w9:string)
  n54 = Transpose 2D Array(2D array=w11) -> (transposed array=w7:string[][])
  n55 = Build Array(w9) -> (w8:string[])
  n56 = call "REPORT.Create Table.vi"("Secction"="0.2# FINAL RESULT TEST ASIC", "Row Headers"=w8, "Text 2d"=w7, "Text In"=w15) -> ("Text Out"=w14:string)  [unwired: 4 in, 1 out]
  n57 = call "REPORT.Create Table.vi"("Secction"="0.3# ASIC TESTING RESULT", "Row Headers"=w19, "Column Headers"=string[] ["REGISTER DEFAULT", "REGISTER W/R", "DEVIATION ADC", "MAX P MIN N", "MIN P MAX N", "RATE SCAN", "RATE SCAN ADDERS", "ANALOG OFFSET", "DIGITAL OFFSET"] ("Row Headers"), "Text 2d"=w20, "Text In"=w14) -> ("Text Out"=w6:string)  [unwired: 3 in, 1 out]
  n58 = Concatenate Strings(w6, "[0.4# NOTES]\nIf not indicated otherwise, ALL values in volts.\nRate Scan & Rate scan Adders: [OUTPUT ASIC] > Values ADC volts (counts ASIC)\nRate Scan Rectified & Rate Scan Adders Rectified [OUTPUT ASIC] > Values ADC volts-Values Offset (Gain)\nDigital Offset & Analog Offset: [OFFSET DETAIL] > Values MIN ADC volts (counts ASIC)/MAX ADC volts (counts ASIC)\n" ("string")) -> (w26:string)
  n59 = call "REPEORT.CAMBIO LINEA.vi"("Text Out"=w26) -> ("String"=→"Text Out":string)  [unwired: 8 in]
